vi "Init.vi"(8 "error in (no error)":errorcluster, 10 "ID":string, 11 "Mixer in":refnum<class "Transport.lvclass">) -> (0 "error out":errorcluster, 3 "Mixer out":refnum<class "Transport.lvclass">)   [LabVIEW 2020, in "Transport.lvclass"]
uses:
  Transport.lvclass
  Transport.lvclass/Transport.ctl
  Packed Libraries/Messaging.lvlibp
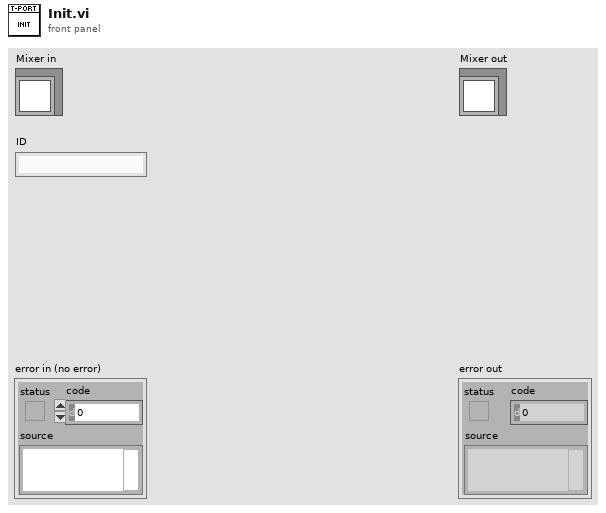
[diagram p1: front panel]
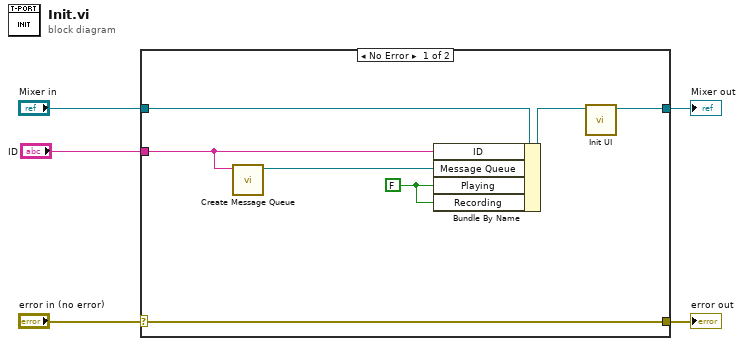
[diagram p0: block diagram]
diagram:
  n1 = case shown="No Error" "error in (no error)" {
    selector: "error in (no error)" -> [w12 w14]
    tunnel: [w12 w14] -> w4
    tunnel: [w7 w13] -> w2
    tunnel: "Mixer in" -> [w11 w13]
    tunnel: "ID" -> [w10 _]
    frame No Error {
      w6 = FALSE ("Playing")
      n2 = call "Create Message Queue.vi"("Queue Name"=w10) -> ("queue out"=w9:refnum<queue>)  [unwired: 9 in, 1 out]
      n3 = Bundle By Name(cluster=w11, "ID"=w10, "Message Queue"=w9, "Playing"=w6, "Recording"=w6) -> (w8:refnum<class "Transport.lvclass">)
      n4 = call "Init UI.vi"("Mixer in"=w8) -> ("Mixer out"=w7:refnum<class "Transport.lvclass">)  [unwired: 9 in, 1 out]
    }
    frame Error {
    }
  }
  "error out" <- w4
  "Mixer out" <- w2
